vi "update volume.vi"(7 "volume id":i32, 8 "error in (no error)":errorcluster, 10 "volume data":T1, 11 "manager_daemon in":refnum<class "manager_daemon.lvclass">) -> (0 "error out":errorcluster, 3 "manager_daemon out":refnum<class "manager_daemon.lvclass">)   [LabVIEW 2024, in "manager_daemon.lvclass"]
uses:
  manager_daemon.lvclass
  type_defs/msg--cluster.ctl
  type_defs/cmd--enum.ctl
  manager_daemon.lvclass/manager_daemon.ctl
  CV_Shared_Library/volume.type--enum.ctl
  CV_Shared_Library/CV_Shared_Library.lvlib
  type_defs/VolumeData--cluster.ctl
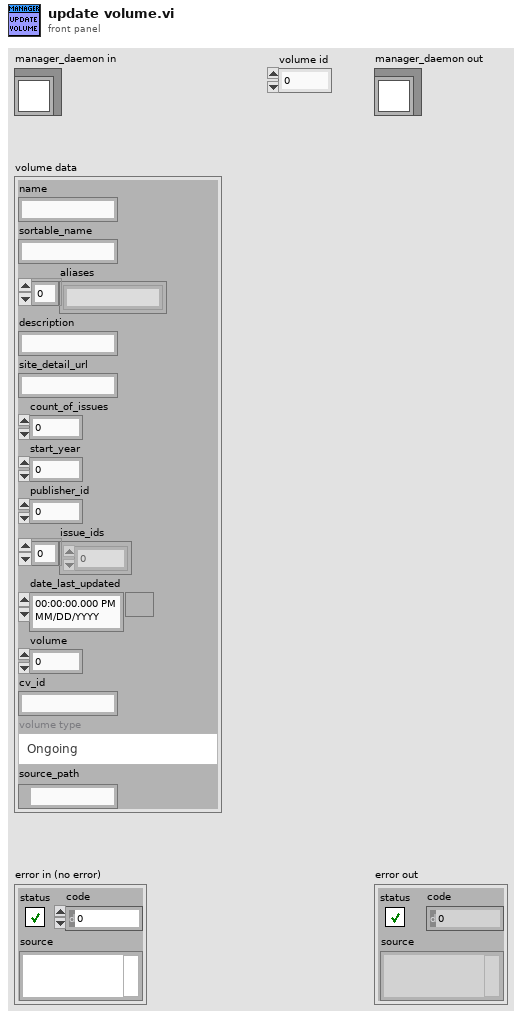
[diagram p1: front panel]
types:
  T1 = typedef "manager_daemon.lvclass/VolumeData--cluster.ctl" = cluster{"name":string, "sortable_name":string, "aliases":string[], "description":string, "site_detail_url":string, "count_of_issues":i32, "start_year":i32, "publisher_id":i32, "issue_ids":i32[], "date_last_updated":timestamp, "volume":i32, "cv_id":string, "volume type":T2, "source_path":path}
  T2 = typedef "CV_Shared_Library.lvlib/volume.type--enum.ctl" = enum16{"Ongoing", "Limited Series", "Annual", "One Shot", "Reprint/Document", "Star Comics", "Epic Comics"}
  T3 = typedef "manager_daemon.lvclass/msg--cluster.ctl" = cluster{"cmd":T4, "data":variant}
  T4 = typedef "manager_daemon.lvclass/cmd--enum.ctl" = enum16{"init", "run", "load binaries", "build binaries", "save binaries", "create folder map", "display info", "apply filter", "add volume", "add issues", "add issue", "get issues", "get volume", "update volume", "delete volume", "delete issues", "exit"}
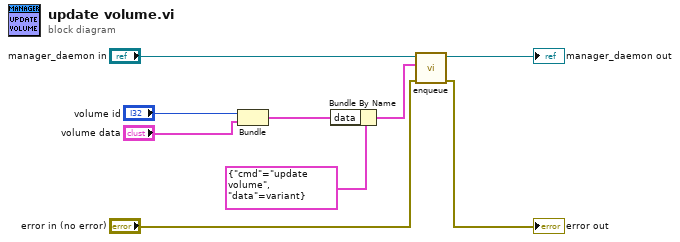
[diagram p0: block diagram]
diagram:
  n1 = Bundle("volume id"="volume id", "volume data"="volume data") -> (w1:cluster{"volume id":i32, "volume data":T1})  [unwired: 1 in]
  n2 = Bundle By Name(cluster=T3 {"cmd"=enum."update volume", "data"=variant} ("msg"), "data"=w1) -> (w6:T3)
  n3 = call "enqueue.vi"("error in (no error)"="error in (no error)", "msg"=w6, "manager_daemon in"="manager_daemon in") -> ("error out"=→"error out":errorcluster, "manager_daemon out"=→"manager_daemon out":refnum<class "manager_daemon.lvclass">)  [unwired: 7 in]
